vi "Konfig AK Paccar.vi"() -> ()   [LabVIEW 2020, in "AK-Schnittstelle.lvlib"]
uses:
  AK-Schnittstelle.lvlib
  Visualisierungs Elemente/VISA Control.ctl
  Seriell - Parity Bits.ctl
  Seriell - Stop Bits.ctl
  Seriell - Flow Control.ctl
  Visualisierungs Elemente/Button.ctl
  Seriell - Baud Rate.ctl
  Seriell - Data Bits.ctl
  Visualisierungs Elemente/String - Ausgabefeld.ctl
  AK Befehlssatz.ctl
  Aktionen Gespeicherte Werte.ctl
  Seiten/FT-IR/FGV FT-IR Gasliste Aktionen.ctl
  AK Namen Aktionen.ctl
  Daten weitergeben Aktionen.ctl
  SysLog/SysLog Interface.ctl
  Seiten/FT-IR/FT-IR.lvlib
  Allgemein/allgemeine Sub-VIs.lvlib
  Sprachverwaltung/Sprachverwaltung.lvlib
  SysLog/SysLog.lvlib
  <vilib>/Utility/Data Type/NI_Data Type.lvlib
  AK Seriell/AK Seriell.lvlib
panel:
  in  "Registerkarte":T1(tab)
  in  "Nur im Messen übertragen":bool caption="Loggen?"
  in  "AK Befehlssatz":T2=enum."AVL (Puma)"
  in  "Timeout":u16
  in  "Loggen?":bool
  in  "data bits":T3=8 items=["8"=8, "7"=7, "6"=6, "5"=5, "4"=4]
  in  "Baud Rate":T4=38400 items=["38400"=38400, "19200"=19200, "14400"=14400, "9600"=9600, "4800"=4800, "2400"=2400]
  in  "TCP aktiv":bool
  in  "Seriell aktiv":bool
  in  "Port":u16
  in  "flow control":T5 items=["None"=0, "XON/XOFF"=1, "RTS/CTS"=2, "DTR/DSR"=4]
  in  "stop bits":T6=10 items=["1.0"=10, "1.5"=15, "2.0"=20]
  in  "parity":T7 items=["None", "Odd", "Even", "Mark", "Space"]
  in  "VISA resource name":T8="COM1"
  in  "Alle Löschen 2":T9 caption="Alle Löschen"
  out "EKFG vom Host":string[](array[string])
  in  "Original Liste":i32(listbox)
  in  "Konfigurierte Liste":i32(listbox)
  in  "Übernehmen":T9
  in  "Löschen":T9
  in  "Alle Löschen":T9
  in  "AK Namen":T10[](array[typedef])
  out "Gasliste":T10[](array[typedef])
  out "Empfangspuffer":string[](array[string])
  out "Antwort":string[](array[string])
  out "Details ALLE":string[](array[string])
  in  "ABBRECHEN":T9
  in  "Speichern":T9
  # "Konfiguration AK-Schnittstelle"
  # "Seriell"
  # "TCP"
  # "Serielle Schnittstelle:"
  # "Port:"
  # "Baud rate:"
  # "Timeout:"
  # "sec"
  # "Data bits:"
  # "Parity bits:"
  # "Stop bits:"
  # "Flow control:"
  # "Messwerte nur in Messen übertragen:"
  # "AK in Datei Loggen:"
  # "AK Befehlssatz:"
  # "Auswahl Gase (EKFG)"
  # "AK Namen vergeben (für EKFG)"
  # "Gasliste"
  # "AK Namen"
  # "Status AK-Kommunikation"
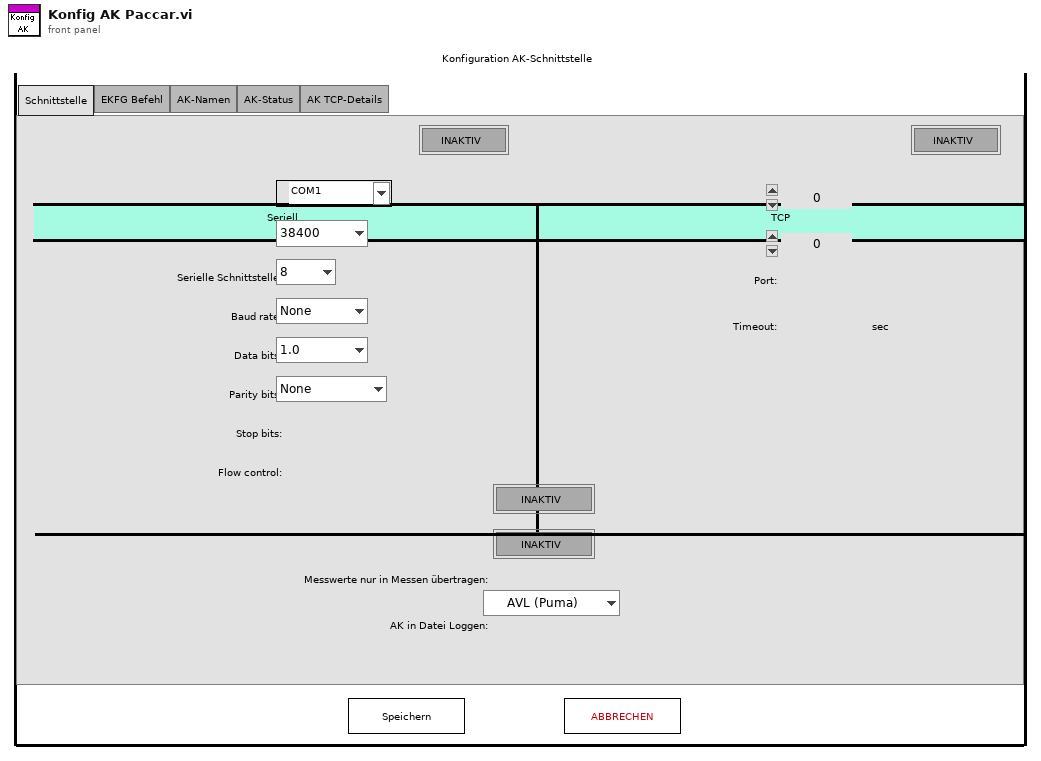
[diagram p1: front panel]
types:
  T1 = enum32{"Interface", "EKFG Commando", "AK-Name", "AK-Status", "AK TCP-Details"}
  T2 = typedef "AK-Schnittstelle.lvlib/AK Befehlssatz.ctl" = enum16{"MEXA", "IAG v1.4", "AVL (Puma)", "PEUS"}
  T3 = typedef "AK-Schnittstelle.lvlib/AK Seriell.lvlib/Seriell - Data Bits.ctl" = u16
  T4 = typedef "AK-Schnittstelle.lvlib/AK Seriell.lvlib/Seriell - Baud Rate.ctl" = u16
  T5 = typedef "AK-Schnittstelle.lvlib/AK Seriell.lvlib/Seriell - Flow Control.ctl" = u16
  T6 = typedef "AK-Schnittstelle.lvlib/AK Seriell.lvlib/Seriell - Stop Bits.ctl" = u16
  T7 = typedef "AK-Schnittstelle.lvlib/AK Seriell.lvlib/Seriell - Parity Bits.ctl" = u16
  T8 = typedef "VISA Control.ctl" = refnum<visa-resource-name>
  T9 = typedef "Button.ctl" = bool
  T10 = typedef "String - Ausgabefeld.ctl" = string
  T11 = typedef "FT-IR.lvlib/FGV FT-IR Gasliste Aktionen.ctl" = enum16{"lesen", "Gasliste FT-IR", "Gasliste ausgelesen", "laden", "speichern", "löschen"}
  T12 = typedef "AK-Schnittstelle.lvlib/AK Namen Aktionen.ctl" = enum16{"lesen", "laden", "speichern Namen", "AK Namen", "Liste erstellen", "EKFG erstellen", "speichern EKFG", "EKFG schreiben", "Neuen Eintrag erzeugen"}
  T13 = typedef "AK-Schnittstelle.lvlib/Aktionen Gespeicherte Werte.ctl" = enum16{"lesen", "laden", "speichern", "Seriell", "TCP", "Diverse", "AKTIV", "AK-Namen"}
  T14 = typedef "AK-Schnittstelle.lvlib/Diverse gespeicherte Werte.ctl" = cluster{"Kalibriergaseingang":i16, "SamplePoint":i16, "CalGas zu PNS":i16, "Gas-Reihenfolge":i16[], "Zeit 0-Gas":sgl, "Zeit CalGas":sgl, "AK Befehlssatz":T2}
  T15 = typedef "AK-Schnittstelle.lvlib/AK TCP.lvlib/TCP Parameter.ctl" = cluster{"Port":u16, "Timeout":u16}
  T16 = typedef "AK-Schnittstelle.lvlib/AK Seriell.lvlib/Serielle Parameter.ctl" = cluster{"VISA resource name":refnum<visa-resource-name>, "baud rate":u32, "data bits":u16, "parity":u16, "stop bits":u16, "flow control":u16}
  T17 = typedef "AK-Schnittstelle.lvlib/Daten weitergeben Aktionen.ctl" = enum16{"lesen", "schreiben", "Log löschen", "Detail", "Detail löschen", "Speicher Freigeben"}
  T18 = typedef "SysLog.lvlib/SysLog Interface.ctl" = cluster{"FehlermeldungsCode":i32, "ErfolgsmeldungsCode":i32, "ParameterListenString":string, "Anzeige":bool, "SysLogIcon":enum16{"OK", "Warnung", "Fehler"}, "intern":bool}
  T19 = typedef "AK-Schnittstelle.lvlib/AK Namen Listen.ctl" = cluster{"Namen":string[], "AK Namen":string[]}
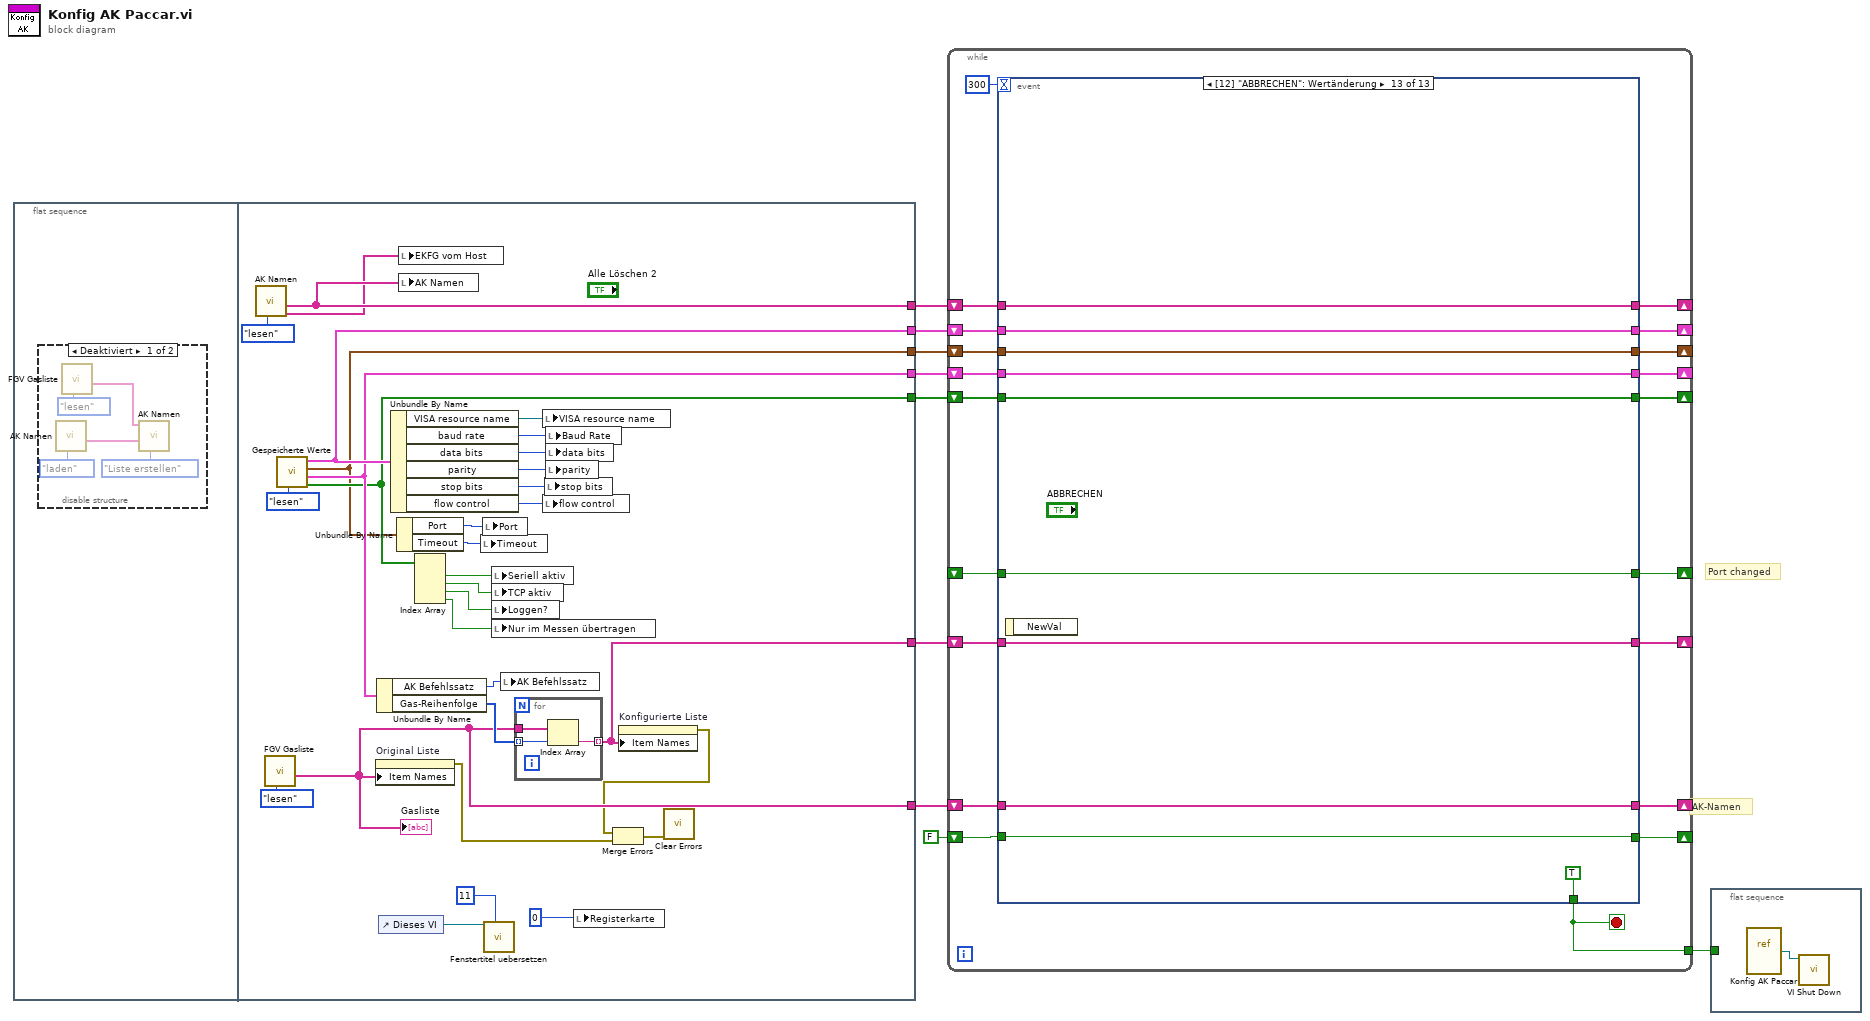
[diagram p0: block diagram]
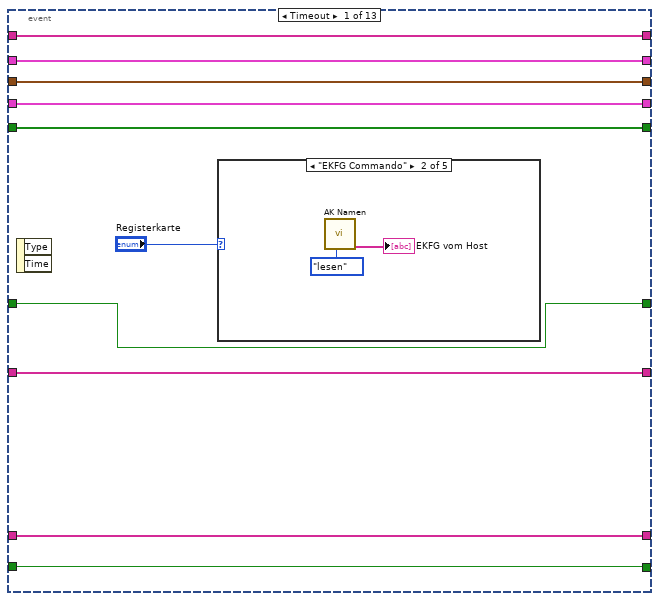
[diagram p3: hidden frame]
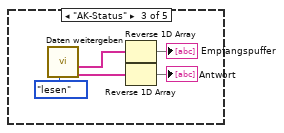
[diagram p5: hidden frame]
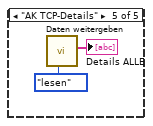
[diagram p7: hidden frame]
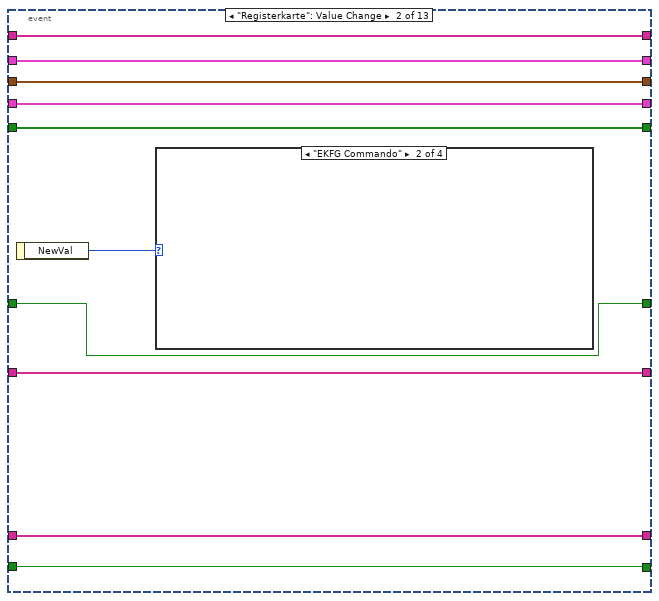
[diagram p8: hidden frame]
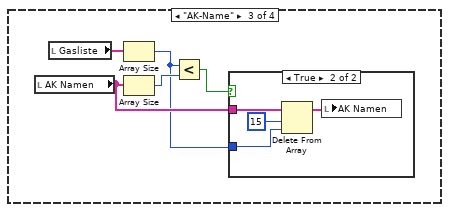
[diagram p10: hidden frame]
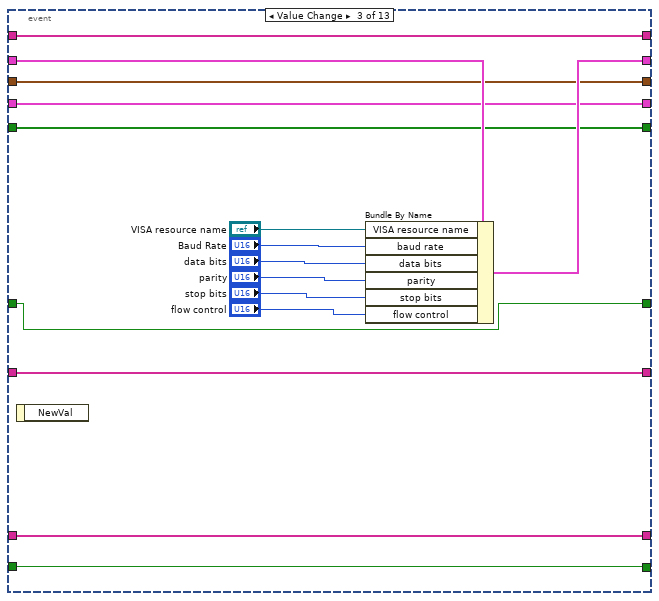
[diagram p13: hidden frame]
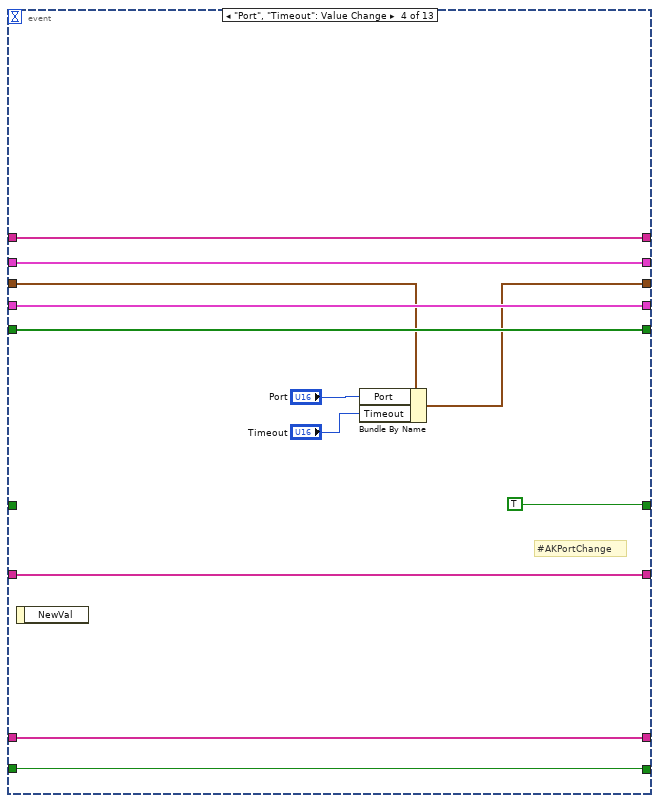
[diagram p14: hidden frame]
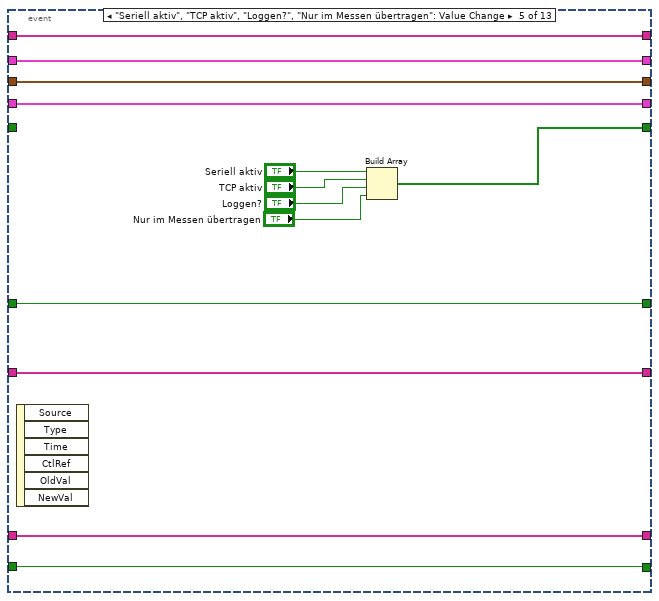
[diagram p15: hidden frame]
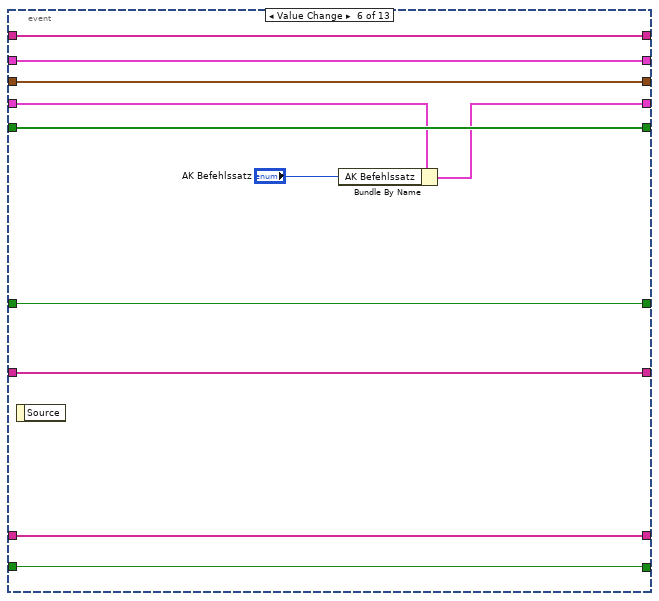
[diagram p16: hidden frame]
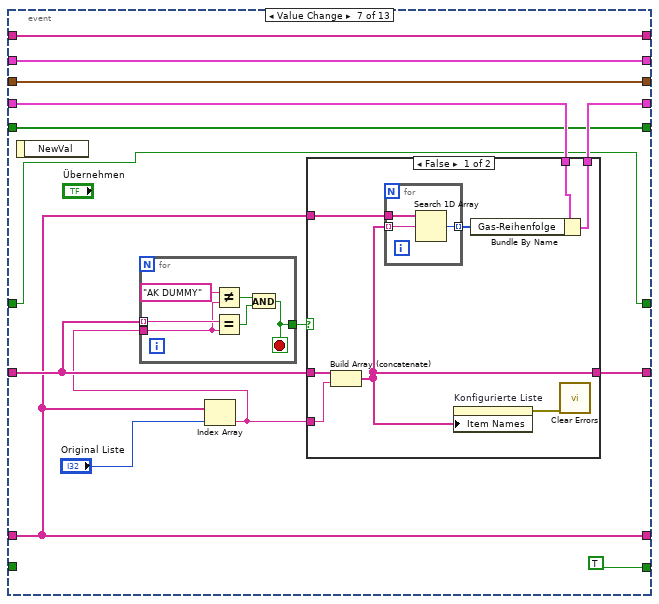
[diagram p17: hidden frame]
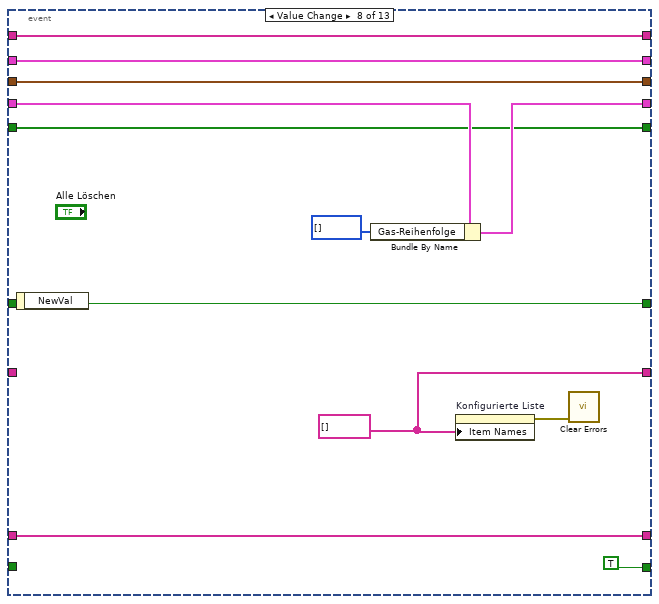
[diagram p19: hidden frame]
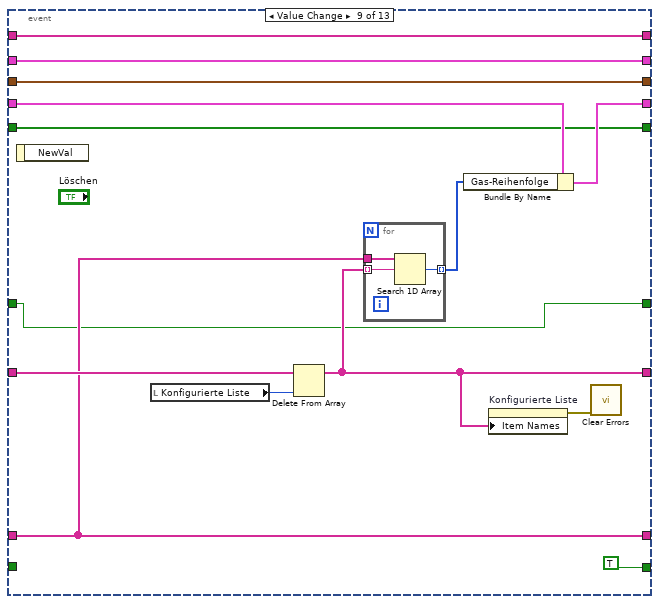
[diagram p20: hidden frame]
diagram:
  # "Port changed"
  # "AK-Namen"
  n1 = flat-sequence {
    tunnel: [w38] -> w9
    tunnel: [w29] -> w8
    tunnel: [w36] -> w7
    tunnel: [w34] -> w6
    tunnel: [w26] -> w4
    tunnel: [w31] -> w5
    tunnel: [w17] -> w3
    frame #0 {
      n2 = disable-structure shown="Deaktiviert" {
        frame Disabled {
          n3 = call "AK Namen.vi"("Aktionen"=AK_Namen_Aktionen."laden") -> ("AK Namen"=w12:string[])  [unwired: 7 in, 3 out]
          n4 = call "FGV Gasliste.vi"("Aktionen"=FGV_FT-IR_Gasliste_Aktionen."lesen") -> ("Aktuelle Gasliste gesamt"=w10:T10[])  [unwired: 8 in, 2 out]
          n5 = call "AK Namen.vi"("Aktionen"=AK_Namen_Aktionen."Liste erstellen", "AK Namen"=w12, "Aktuelle Gasliste FT-IR"=w10) -> ()  [unwired: 5 in, 4 out]
        }
        frame Enabled {
        }
      }
    }
    frame #1 {
      n6 = call "AK Namen.vi"("Aktionen"=AK_Namen_Aktionen."lesen") -> ("EKFG Liste"=w16:string[], "AK Namen"=w17:string[])  [unwired: 7 in, 2 out]
      n7 = call "FGV Gasliste.vi"("Aktionen"=FGV_FT-IR_Gasliste_Aktionen."lesen") -> ("Aktuelle Gasliste gesamt"=w26:T10[])  [unwired: 8 in, 2 out]
      "Gasliste" <- w26
      n8 = call "Gespeicherte Werte.vi"("Aktionen"=Aktionen_Gespeicherte_Werte."lesen") -> ("AKTIV?"=w31:bool[], "Diverse Werte"=w36:T14, "TCP Parameter"=w29:T15, "Serielle Parameter"=w38:T16)  [unwired: 6 in, 1 out]
      n9 = property on="Original Liste" class="Listenfeld (strikt)"("Item Names"=w26) -> (error out=w23:errorcluster)  [unwired: 2 in, 1 out]
      n10 = Unbundle By Name(w36) -> ("AK Befehlssatz"=w25:T2, "Gas-Reihenfolge"=w35:i16[])
      n11 = control-ref of="Dieses VI"() -> (w20:refnum<vi>)
      n12 = Unbundle By Name(w38) -> ("VISA resource name"=w44:refnum<visa-resource-name>, "baud rate"=w43:u32, "data bits"=w42:u16, "parity"=w41:u16, "stop bits"=w40:u16, "flow control"=w39:u16)
      n13 = Unbundle By Name(w29) -> ("Port"=w28:u16, "Timeout"=w27:u16)
      n14 = local write "EKFG vom Host"(w16) -> ()
      n15 = local write "AK Namen"(w17) -> ()
      n16 = Index Array(array=w31) -> (element #1=w33:bool, element #2=w32:bool, element #3=w30:bool, element #4=w21:bool)  [unwired: 4 in]
      n17 = local write "Timeout"(w27) -> ()
      n18 = local write "Port"(w28) -> ()
      n19 = call "Fenstertitel uebersetzen.vi"("Index (Seite)"=11, "Dieses VI"=w20) -> ()  [unwired: 8 in, 2 out]
      n20 = local write "Seriell aktiv"(w33) -> ()
      n21 = local write "TCP aktiv"(w32) -> ()
      n22 = local write "Loggen?"(w30) -> ()
      n23 = local write "Nur im Messen übertragen"(w21) -> ()
      n24 = local write "AK Befehlssatz"(w25) -> ()
      n25 = for {
        tunnel: w35 -> [w48] mode=indexing
        tunnel: w26 -> [w47]
        tunnel: [w46] -> w34 mode=indexing
        n26 = Index Array(array=w47, index=w48) -> (element=w46:T10)
      }
      n27 = local write "VISA resource name"(w44) -> ()
      n28 = local write "flow control"(w39) -> ()
      n29 = local write "stop bits"(w40) -> ()
      n30 = local write "Baud Rate"(w43) -> ()
      n31 = local write "data bits"(w42) -> ()
      n32 = local write "parity"(w41) -> ()
      n33 = local write "Registerkarte"(0) -> ()
      n34 = property on="Konfigurierte Liste" class="Listenfeld (strikt)"("Item Names"=w34) -> (error out=w24:errorcluster)  [unwired: 2 in, 1 out]
      n35 = Merge Errors(w24, w23) -> (w22:errorcluster)
      n36 = call <vilib>:"Clear Errors.vi"("error in (no error)"=w22) -> ()  [unwired: 5 in, 2 out]
    }
  }
  n37 = while {
    shift-right: [w66] -> _
    shift-left: w9 -> [w67]
    shift-right: [w63] -> _
    shift-left: w8 -> [w65]
    shift-right: [w62] -> _
    shift-left: w7 -> [w64]
    shift-right: [w60] -> _
    shift-left: w6 -> [w61]
    shift-right: [w58] -> _
    shift-left: w5 -> [w59]
    shift-right: [w57] -> _
    shift-left: w4 -> [w56]
    shift-right: [w54] -> _
    shift-left: w3 -> [w55]
    tunnel: [w53] -> w2
    shift-right: [w52] -> _
    shift-left: FALSE -> [w51]
    shift-right: [w50] -> _
    shift-left: _ -> [w49]
    stop <- w53 stop-if-true
    n38 = event shown="[12] \"ABBRECHEN\": Wertänderung" {
      selector: _ -> [_ _ _ _ _ _ _ _ _ _ _ _ _]
      dyn-events: _ -> [_ _ _ _ _ _ _ _ _ _ _ _ _]
      timeout: 300 -> [_ _ _ _ _ _ _ _ _ _ _ _ _]
      tunnel: w67 -> [w78 w93 w122 w134 w144 w157 w172 w203 w217 w232 w249 w279 w305]
      tunnel: [w78 w93 w121 w134 w144 w157 w172 w203 w217 w232 w249 w279 w305] -> w66
      tunnel: [_ _ _ _ _ _ _ _ _ _ _ TRUE ("ABBRECHEN") TRUE ("ABBRECHEN")] -> w53
      tunnel: w65 -> [w77 w92 w115 w129 w143 w156 w171 w202 w216 w231 w248 w278 w303]
      tunnel: w64 -> [w76 w91 w116 w133 w142 w152 w168 w199 w213 w229 w247 w259 w302]
      tunnel: [w77 w92 w115 w126 w143 w156 w171 w202 w216 w231 w248 w278 w303] -> w63
      tunnel: [w76 w91 w116 w133 w142 w150 w167 w198 w212 w228 w247 w259 w302] -> w62
      tunnel: w61 -> [w70 w96 w114 w132 w145 w154 w166 _ w215 _ w245 w273 w301]
      tunnel: [w70 w96 w114 w132 w145 w154 w169 w201 w211 w227 w245 w273 w301] -> w60
      tunnel: w59 -> [w75 w90 w113 w131 _ w155 w163 w197 w209 w226 w246 w270 w300]
      tunnel: [w75 w90 w113 w131 w141 w155 w163 w197 w209 w226 w246 w270 w300] -> w58
      tunnel: [w73 w95 w110 w130 w140 w153 w162 w196 w208 w225 w244 w269 w299] -> w57
      tunnel: w56 -> [w73 w95 w110 w130 w140 w153 w162 w196 w208 w225 w244 w269 w299]
      tunnel: w55 -> [w72 w94 w109 w125 w138 w158 w161 w195 w207 w224 _ w267 w298]
      tunnel: [w72 w94 w109 w125 w138 w158 w161 w195 w207 w224 w238 w267 w298] -> w54
      tunnel: [w71 w89 w108 w124 w136 w149 TRUE TRUE TRUE TRUE w237 w262 w297] -> w52
      tunnel: w51 -> [w71 w89 w108 w124 w136 w149 _ _ _ _ w237 w262 w297]
      tunnel: [w69 w88 w107 TRUE w135 w148 w159 w192 w204 w221 w236 FALSE w296] -> w50
      tunnel: w49 -> [w69 w88 w107 _ w135 w148 w159 w192 w204 w221 w236 w255 w296]
      event Timeout {
        n39 = event-data() -> ()  [unwired: 1 in, 2 out]
        n40 = case shown="\"EKFG Commando\"" "Registerkarte" {
          frame "Interface", Default {
          }
          frame "EKFG Commando" {
            n41 = call "AK Namen.vi"("Aktionen"=AK_Namen_Aktionen."lesen") -> ("EKFG Liste"=→"EKFG vom Host":string[])  [unwired: 7 in, 3 out]
          }
          frame "AK-Status" {
            n42 = call "Daten weitergeben.vi"("Aktionen"=Daten_weitergeben_Aktionen."lesen") -> ("Antwort"=w82:string[], "Empfangspuffer"=w84:string[])  [unwired: 6 in, 3 out]
            n43 = Reverse 1D Array(array=w84) -> (reversed array=→"Empfangspuffer":string[])
            n44 = Reverse 1D Array(array=w82) -> (reversed array=→"Antwort":string[])
          }
          frame "AK-Name" {
          }
          frame "AK TCP-Details" {
            n45 = call "Daten weitergeben.vi"("Aktionen"=Daten_weitergeben_Aktionen."lesen") -> ("Details ALLE"=→"Details ALLE":string[])  [unwired: 6 in, 4 out]
          }
        }
      }
      event "Registerkarte": Value Change {
        n46 = event-data() -> ("NewVal"=w97:T1)  [unwired: 1 in]
        n47 = case shown="\"EKFG Commando\"" w97 {
          frame "Interface", Default {
          }
          frame "EKFG Commando" {
          }
          frame "AK-Name" {
            n48 = local read "AK Namen"() -> (w100:T10[])
            n49 = local read "Gasliste"() -> (w102:T10[])
            n50 = Array Size(array=w102) -> (size(s)=w99:i32)
            n51 = Array Size(array=w100) -> (size(s)=w101:i32)
            n52 = Less?(x=w99, y=w101) -> (x < y?=w98:bool)
            n53 = case shown="True" w98 {
              tunnel: w100 -> [_ w106]
              tunnel: w99 -> [_ w103]
              frame False {
              }
              frame True {
                n54 = Delete From Array(array=w106, length=15 ("Länge"), index=w103) -> (array with subset deleted=w104:T10[])  [unwired: 1 out]
                n55 = local write "AK Namen"(w104) -> ()
              }
            }
          }
          frame "AK-Status" {
          }
        }
      }
      event Value Change {
        n56 = event-data() -> ()  [unwired: 1 in, 1 out]
        n57 = Bundle By Name(cluster=w122, "VISA resource name"="VISA resource name", "baud rate"="Baud Rate", "data bits"="data bits", "parity"="parity", "stop bits"="stop bits", "flow control"="flow control") -> (w121:T16)
      }
      event "Port", "Timeout": Value Change {
        # "#AKPortChange"
        n58 = event-data() -> ()  [unwired: 1 in, 1 out]
        n59 = Bundle By Name(cluster=w129, "Port"="Port", "Timeout"="Timeout") -> (w126:T15)
      }
      event "Seriell aktiv", "TCP aktiv", "Loggen?", "Nur im Messen übertragen": Value Change {
        n60 = event-data() -> ()  [unwired: 1 in, 6 out]
        n61 = Build Array("Seriell aktiv", "TCP aktiv", "Loggen?", "Nur im Messen übertragen") -> (w141:bool[])
      }
      event Value Change {
        n62 = event-data() -> ()  [unwired: 1 in, 1 out]
        n63 = Bundle By Name(cluster=w152, "AK Befehlssatz"="AK Befehlssatz") -> (w150:T14)
      }
      event Value Change {
        n64 = event-data() -> ()  [unwired: 1 in, 1 out]
        n65 = Index Array(array=w162, index="Original Liste") -> (element=w165:T10)
        n66 = for {
          tunnel: w166 -> [w178] mode=indexing
          tunnel: w165 -> [w177]
          tunnel: [w173] -> w164
          stop <- w173 stop-if-true
          n67 = Not Equal?(x="AK DUMMY", y=w177) -> (x != y?=w175:bool)
          n68 = Equal?(x=w178, y=w177) -> (x = y?=w174:bool)
          n69 = And(x=w175, y=w174) -> (x .and. y?=w173:bool)
        }
        n70 = case shown="False" w164 {
          tunnel: w166 -> [w186 w190]
          tunnel: w165 -> [w185 _]
          tunnel: w162 -> [w184 _]
          tunnel: [w183 w190] -> w169
          tunnel: w168 -> [w182 w191]
          tunnel: [w181 w191] -> w167
          frame False {
            n71 = Build Array (concatenate)(w186, w185) -> (w183:T10[])
            n72 = for {
              tunnel: w184 -> [w189]
              tunnel: w183 -> [w188] mode=indexing
              tunnel: [w187] -> w180 mode=indexing
              n73 = Search 1D Array(1D array=w189, element=w188) -> (index of element=w187:i32)  [unwired: 1 in]
            }
            n74 = property on="Konfigurierte Liste" class="Listenfeld (strikt)"("Item Names"=w183) -> (error out=w179:errorcluster)  [unwired: 2 in, 1 out]
            n75 = Bundle By Name(cluster=w182, "Gas-Reihenfolge"=w180) -> (w181:T14)
            n76 = call <vilib>:"Clear Errors.vi"("error in (no error)"=w179) -> ()  [unwired: 5 in, 2 out]
          }
          frame True {
          }
        }
      }
      event Value Change {
        w201 = string[] [] ("Objektnamen")
        n77 = event-data() -> ()  [unwired: 1 in, 1 out]
        n78 = Bundle By Name(cluster=w199, "Gas-Reihenfolge"=i16[] []) -> (w198:T14)
        n79 = property on="Konfigurierte Liste" class="Listenfeld (strikt)"("Item Names"=w201) -> (error out=w194:errorcluster)  [unwired: 2 in, 1 out]
        n80 = call <vilib>:"Clear Errors.vi"("error in (no error)"=w194) -> ()  [unwired: 5 in, 2 out]
      }
      event Value Change {
        n81 = event-data() -> ()  [unwired: 1 in, 1 out]
        n82 = local read "Konfigurierte Liste"() -> (w210:i32)
        n83 = Delete From Array(array=w215, index=w210) -> (array with subset deleted=w211:T10[])  [unwired: 1 in, 1 out]
        n84 = for {
          tunnel: w208 -> [w220]
          tunnel: w211 -> [w219] mode=indexing
          tunnel: [w218] -> w214 mode=indexing
          n85 = Search 1D Array(1D array=w220, element=w219) -> (index of element=w218:i32)  [unwired: 1 in]
        }
        n86 = Bundle By Name(cluster=w213, "Gas-Reihenfolge"=w214) -> (w212:T14)
        n87 = property on="Konfigurierte Liste" class="Listenfeld (strikt)"("Item Names"=w211) -> (error out=w206:errorcluster)  [unwired: 2 in, 1 out]
        n88 = call <vilib>:"Clear Errors.vi"("error in (no error)"=w206) -> ()  [unwired: 5 in, 2 out]
      }
      event "Konfigurierte Liste": Drag Ended {
        n89 = event-data() -> ()  [unwired: 1 in, 1 out]
        n90 = property on="Konfigurierte Liste" class="Listenfeld (strikt)"() -> (error out=w223:errorcluster, "Item Names"=w227:string[])  [unwired: 2 in, 1 out]
        n91 = call <vilib>:"Clear Errors.vi"("error in (no error)"=w223) -> ()  [unwired: 5 in, 2 out]
        n92 = for {
          tunnel: w225 -> [w235]
          tunnel: w227 -> [w234] mode=indexing
          tunnel: [w233] -> w230 mode=indexing
          n93 = Search 1D Array(1D array=w235, element=w234) -> (index of element=w233:i32)  [unwired: 1 in]
        }
        n94 = Bundle By Name(cluster=w229, "Gas-Reihenfolge"=w230) -> (w228:T14)
      }
      event "AK Namen": Value Change {
        n95 = event-data() -> ()  [unwired: 1 in, 1 out]
        n96 = local read "Gasliste"() -> (w243:T10[])
        n97 = Array Size(array=w243) -> (size(s)=w241:i32)
        n98 = Array Size(array="AK Namen") -> (size(s)=w242:i32)
        n99 = Less?(x=w241, y=w242) -> (x < y?=w240:bool)
        n100 = case shown="True" w240 {
          tunnel: "AK Namen" -> [w250 w254]
          tunnel: w241 -> [_ w252]
          tunnel: [w250 w251] -> w238
          frame False {
          }
          frame True {
            n101 = Delete From Array(array=w254, length=15 ("Länge"), index=w252) -> (array with subset deleted=w251:T10[])  [unwired: 1 out]
            n102 = local write "AK Namen"(w251) -> ()
          }
        }
      }
      event Value Change {
        # "AK-Namen"
        n103 = event-data() -> ()  [unwired: 1 in, 1 out]
        n104 = call "Gespeicherte Werte.vi"("Aktionen"=Aktionen_Gespeicherte_Werte."Seriell", "Serielle Parameter"=w279) -> ("Serielle Parameter"=w275:T16)  [unwired: 5 in, 4 out]
        n105 = Unbundle By Name(w259) -> ("AK Befehlssatz"=w257:T2)
        n106 = case shown="True" w262 {
          frame False {
          }
          frame True {
            n107 = stacked-sequence {
              frame #0 {
                n108 = call "AK Namen.vi"("Aktionen"=AK_Namen_Aktionen."EKFG schreiben") -> ()  [unwired: 7 in, 4 out]
              }
              frame #1 {
                n109 = call "AK Namen.vi"("Aktionen"=AK_Namen_Aktionen."speichern EKFG") -> ()  [unwired: 7 in, 4 out]
              }
            }
          }
        }
        n110 = call "Gespeicherte Werte.vi"("Port changed in"=w255, "Aktionen"=Aktionen_Gespeicherte_Werte."TCP", "TCP Parameter"=w278, "Serielle Parameter"=w275) -> ("Diverse Werte"=w260:T14, "Serielle Parameter"=w274:T16)  [unwired: 3 in, 3 out]
        n111 = Unbundle By Name(w260) -> ("AK Befehlssatz"=w261:T2)
        n112 = call "Gespeicherte Werte.vi"("Aktionen"=Aktionen_Gespeicherte_Werte."Diverse", "Diverse Werte"=w259, "Serielle Parameter"=w274) -> ("Serielle Parameter"=w271:T16)  [unwired: 4 in, 4 out]
        n113 = Not Equal?(x=w261, y=w257) -> (x != y?=w258:bool)
        n114 = case shown="True" w258 {
          tunnel: w257 -> [_ w283]
          frame False {
          }
          frame True {
            n115 = disable-structure shown="SysLogAktiv==TRUE" {
              disable-tunnel: w283 -> [w290 _]
              frame condition #0 (active) {
                n116 = call <vilib>:"Get Numeric Information.vi"("variant"=AK_Befehlssatz."IAG v1.4" ("AK Befehlssatz")) -> ("enum names"=w289:string[])  [unwired: 7 in, 3 out]
                n117 = Index Array(array=w289, index=w290) -> (element=w284:string)
                n118 = Bundle By Name(cluster=T18 {"FehlermeldungsCode"=9, "ErfolgsmeldungsCode"=9, "ParameterListenString"="", "Anzeige"=TRUE, "SysLogIcon"=enum."OK", "intern"=FALSE} ("Cluster (in)"), "ParameterListenString"=w284) -> (w285:T18)
                n119 = call "Syslog Interface PC.vi"("Fehler (in)"=errorcluster {"status"=FALSE, "code"=0, "source"=""}, "Cluster (in)"=w285) -> ()  [unwired: 9 in, 1 out]
              }
              frame condition #1 {
              }
            }
          }
        }
        n120 = call "Gespeicherte Werte.vi"("Aktionen"=Aktionen_Gespeicherte_Werte."AKTIV", "AKTIV?"=w270, "Serielle Parameter"=w271) -> ("Serielle Parameter"=w268:T16)  [unwired: 4 in, 4 out]
        n121 = flat-sequence {
          tunnel: w264 -> [_]
          frame #0 {
            n122 = call "FGV Gasliste.vi"("Aktionen"=FGV_FT-IR_Gasliste_Aktionen."lesen") -> ("Aktuelle Gasliste gesamt"=w293:T10[])  [unwired: 8 in, 2 out]
            n123 = call "AK Namen.vi"("Aktionen"=AK_Namen_Aktionen."Liste erstellen", "Aktuelle Gasliste FT-IR"=w293) -> ()  [unwired: 6 in, 4 out]
          }
        }
        n124 = call "AK Namen.vi"("Aktionen"=AK_Namen_Aktionen."AK Namen", "AK Namen"=w267) -> ("Namen"=w266:string[])  [unwired: 6 in, 3 out]
        n125 = call "Gespeicherte Werte.vi"("Aktionen"=Aktionen_Gespeicherte_Werte."speichern", "Serielle Parameter"=w268) -> ()  [unwired: 5 in, 5 out]
        n126 = call "AK Namen.vi"("Aktionen"=AK_Namen_Aktionen."speichern Namen", "Aktuelle Gasliste FT-IR"=w266) -> ("AK Namen Liste"=w264:T19)  [unwired: 6 in, 3 out]
      }
      event Value Change {
        n127 = event-data() -> ()  [unwired: 1 in, 1 out]
      }
    }
  }
  n128 = flat-sequence {
    tunnel: w2 -> [_]
    frame #0 {
      n129 = vi-ref "Konfig AK Paccar.vi"() -> (w306:refnum<vi>)
      n130 = call "VI Shut Down.vi"("VI Referenz"=w306) -> ()  [unwired: 11 in]
    }
  }
